vi "Launch Batch Processor.vi"() -> ()   [LabVIEW 2016]
uses:
  Batch Processor.lvclass
  C:/github/LabActor/Controllers/Application Controller/Application Controller.lvclass
  Application Controller/Load App.vi
  Application Controller/Application Controller.lvclass
panel:
  out "Waiting Lights":T1
  out "Current action:":string
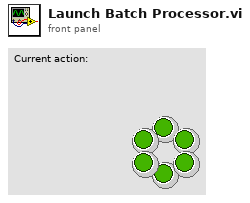
[diagram p1: front panel]
types:
  T1 = cluster{"DNL_wait 1":bool, "DNL_wait 1":bool, "DNL_wait 1":bool, "DNL_wait 1":bool, "DNL_wait 1":bool, "DNL_wait 1":bool}
  T2 = cluster{"[0]":bool, "[1]":bool, "[2]":bool, "[3]":bool, "[4]":bool, "[5]":bool}
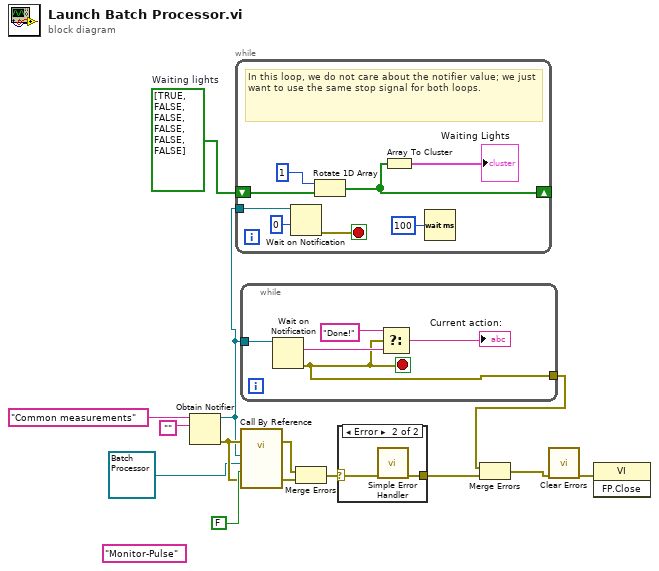
[diagram p0: block diagram]
diagram:
  (unwired) "Monitor-Pulse" ("Name")
  w3 = bool[] [TRUE, FALSE, FALSE, FALSE, FALSE, FALSE]  # Waiting lights
  n1 = Obtain Notifier(name (unnamed)="Common measurements", notification data type="") -> (notifier out=w2:refnum<notifier>, error out=w9:errorcluster)  [unwired: 2 in, 1 out]
  n2 = while {
    shift-right: [w16] -> _
    shift-left: w3 -> [w18]
    tunnel: w2 -> [w20]
    stop <- w22 stop-if-true
    # "In this loop, we do not care about the notifier value; we just want to use the same stop signal for both loops."
    n3 = Wait on Notification(notifier=w20, timeout in ms (-1)=0) -> (error out=w22:errorcluster)  [unwired: 2 in, 3 out]
    n4 = Rotate 1D Array(1:w18, 2:1 ("n")) -> (0:w16:bool[])
    n5 = Array To Cluster(array=w16) -> (cluster=→"Waiting Lights":T2)
    n6 = Wait (ms)(milliseconds to wait=u32 100) -> ()  [unwired: 1 out]
  }
  n7 = while {
    tunnel: w2 -> [w27]
    tunnel: [w23] -> w4
    stop <- w23 stop-if-true
    n8 = Wait on Notification(notifier=w27) -> (notification=w25:string, error out=w23:errorcluster)  [unwired: 3 in, 2 out]
    n9 = Select(t="Done!" ("notification"), s=w23, f=w25) -> (s? t:f=→"Current action:":string)
  }
  n10 = call-by-ref "?"(error in=w9, "Error In"=w9, "Open Actor Core front panel? (F)"=FALSE, "Application Controller.lvclass"=refnum<class "Batch Processor.lvclass"> refnum ("Batch Processor.lvclass"), "Status Notifier"=w2) -> (error out=w12:errorcluster, "Error Out"=w8:errorcluster)  [unwired: 8 in, 1 out]
  n11 = Merge Errors(w12, w8) -> (w13:errorcluster)
  n12 = case shown="Error" w13 {
    selector: w13 -> [w28 w30]
    tunnel: [w28 w29] -> w6
    frame No Error {
    }
    frame Error {
      n13 = call <vilib>:"Simple Error Handler.vi"("error in (no error)"=w30) -> ("error out"=w29:errorcluster)  [unwired: 4 in, 4 out]
    }
  }
  n14 = Merge Errors(w4, w6) -> (w5:errorcluster)
  n15 = call <vilib>:"Clear Errors.vi"("error in (no error)"=w5) -> ("error out"=w14:errorcluster)  [unwired: 5 in, 1 out]
  n16 = invoke class="VI" method="FP.Close"(error in=w14) -> ()  [unwired: 2 in, 3 out]
